vi "Create_Trajectory_Using_PathfinderSwerve_NAT.vi"() -> ()   [LabVIEW 2019]
uses:
  <vilib>/Rock Robotics/WPI/ThirdParty/JAS_Junk/JaciPathFinderLib/VIs/Waypoint.ctl
  <vilib>/Rock Robotics/WPI/ThirdParty/JAS_Junk/TrajLib/TRAJ_STATE.ctl
  <vilib>/Rock Robotics/WPI/ThirdParty/JAS_Junk/TrajLib/POSE2D.ctl
  <vilib>/Rock Robotics/WPI/ThirdParty/JAS_Junk/TrajLib/TRANSLATION2D.ctl
  <vilib>/Rock Robotics/WPI/ThirdParty/JAS_Junk/TrajLib/ROTATION2D.ctl
  <vilib>/Rock Robotics/WPI/ThirdParty/JAS_Junk/TrajLib/UTIL_PATHFINDER_CONFIG.ctl
  <vilib>/Rock Robotics/WPI/ThirdParty/JAS_Junk/TrajLib/DISPLAY_WAYPOINT.ctl
  <vilib>/Utility/inputDevices.llb/mouseAcquire.vi
  <vilib>/Rock Robotics/WPI/ThirdParty/JAS_Junk/JaciPathFinderLib/Pathfinder.lvlib
  <vilib>/Rock Robotics/WPI/ThirdParty/JAS_Junk/TrajLib/Trajectory_Library.lvlib
panel:
  out "Scrolling":i32
  out "Cursor Update Mode":i32=1
  out "Index":i32
  out "Angle":dbl
  out "CursIdx":i32
  in  "End Program":bool
  in  "Tab Control":T1(tab)
  in  "max_velocity":dbl=58.0
  in  "max_acceleration":dbl=65.0
  in  "max_jerk":dbl=70.0
  in  "wheelbase_width":dbl=20.866
  in  "Real max\n speed":dbl=65.0
  in  "wheelbase_depth":dbl=28.0
  in  "mode":u32(ring) items=["SWERVE_DEFAULT"]
  out "Position":cluster{dbl[], dbl[]}[](graph)
  in  "Remove Cursor":bool
  in  "Add Cursor":bool
  in  "Waypoints":T2[](array[typedef])=[{"x"=15.0, "y"=105.0, "angle"=-45.0}, {"x"=105.0, "y"=65.0, "angle"=0.0}, {"x"=210.0, "y"=106.0, "angle"=45.0}]
  in  "Path Results\ndT":dbl=0.02 format="%7.3f"
  in  "sample_count":i32=100000
  out "Path calculation error":errorcluster
  in  "Calculate\nPath":bool
  out "Complete,\nReady to \nSave file":bool
  out "Path \nSpeed > \nMax":bool
  out "max speed":dbl
  out "Path Data":cluster{dbl[], dbl[]}[](graph)
  out "Traj States\nSize":i32
  out "Trajectory States":T3[](array[typedef]) {"POSE"."ROTATION"."SIN" format="%13.4f"; "POSE"."ROTATION"."COS" format="%13.4f"; "POSE"."ROTATION"."VALUE" format="%13.4f"; "POSE"."TRANSLATION"."Y" format="%14.3f"; "POSE"."TRANSLATION"."X" format="%14.3f"}
  out "File Saved\nWithout\nError":bool
  in  "Trajectory Type":enum32{"Radio Selection 1", "Radio Selection 2"}(radio)
  out "File Creation\nError":errorcluster
  in  "Trajectory File Comment":string
  in  "Trajectory File Name":path
  in  "CreateCmdList":bool
  # "Create trajectory using \"Jaci's Pathfinder\"  (Display for swerve drive robot)"
  # "Instructions:\n----------------  \nThis utility will create a trajectory,, show the data on the various tabs, and optionally write a \"robot relative\" trajectory to a \nfile. To use this utility:\n\n1) Read all of these instructions!\n2) Define the Robot Data. on the \"Robot Data\" tab.\n3) Define the \"Path Definition\" on the \"Define / Create Trajectory\" tab.  These are the beginning and ending positions/headings, and \n     internal positions/headings.\n4) Define the time increment.  0.020 is chosen since that matches the normal robot loop time.\n5) Define \"sample count\".  This is an internal PathFinder variable.  Leaving the value as default should work correctly.  Making \n    the value a little smaller will speed the program up a little.\n6) Press the \"Calculate Path\".  If a good path was calculated it will be displayed on the \"Field Position tab, and the \"Complete, \n    Ready to Save\" indicator will light.  The path can be recalculated many times before performing any other action.\n\nAfter a Path has been calculated, the \"trajectory can be written to a file.  The absolute path is converted to a robot relative \ntrajectory.  To do this:\n1) Enter a comment to be included in the file.  Anything can be entered.\n2) Select the file name.\n3) Select the type of trajectory to save, absolute or relative.\n4) Press \"Create Trajectory File\"  If an error occurs it will be displayed in the File Creation Error indicator.\n\nNotes:\n---------\n- All the robot parameters, path, and field dimensions are in INCHES, and DEGREES.  The resulting trajectory is converted to \n   METERS, and RADIANS to match the rest of this library!\n- The pathfinder path generation logic doesn't account distribution of speed to the left and right wheels.  As a result the \n   maximum speed can be exceeded.If this happens, but Path Speed > Max light will light and Ready to Execute will not \n   light.  Lower the maximum speed in the Robot Data tab and recalulate the path.  (CURRENTLY THIS LOGIC IS NOT COMPLETE.)\n- 2019 playing field size - width: 26 ft 11.25 In = 323.25 in , length: 52 ft 5.25 in = 629.25 in  (I didn't verify this for the 2020 version.)"
  # "ROBOT DATA"
  # "INCHES/SEC"
  # "INCHES/SEC"
  # "INCHES/SEC^2"
  # "INCHES/SEC^3"
  # "Simulated robot wheelbase is: 20.866"
  # "INCHES"
  # "Simulated robot max speed is: 68.266"
  # "INCHES"
  # "SEC"
  # "PATH DEFINITION"
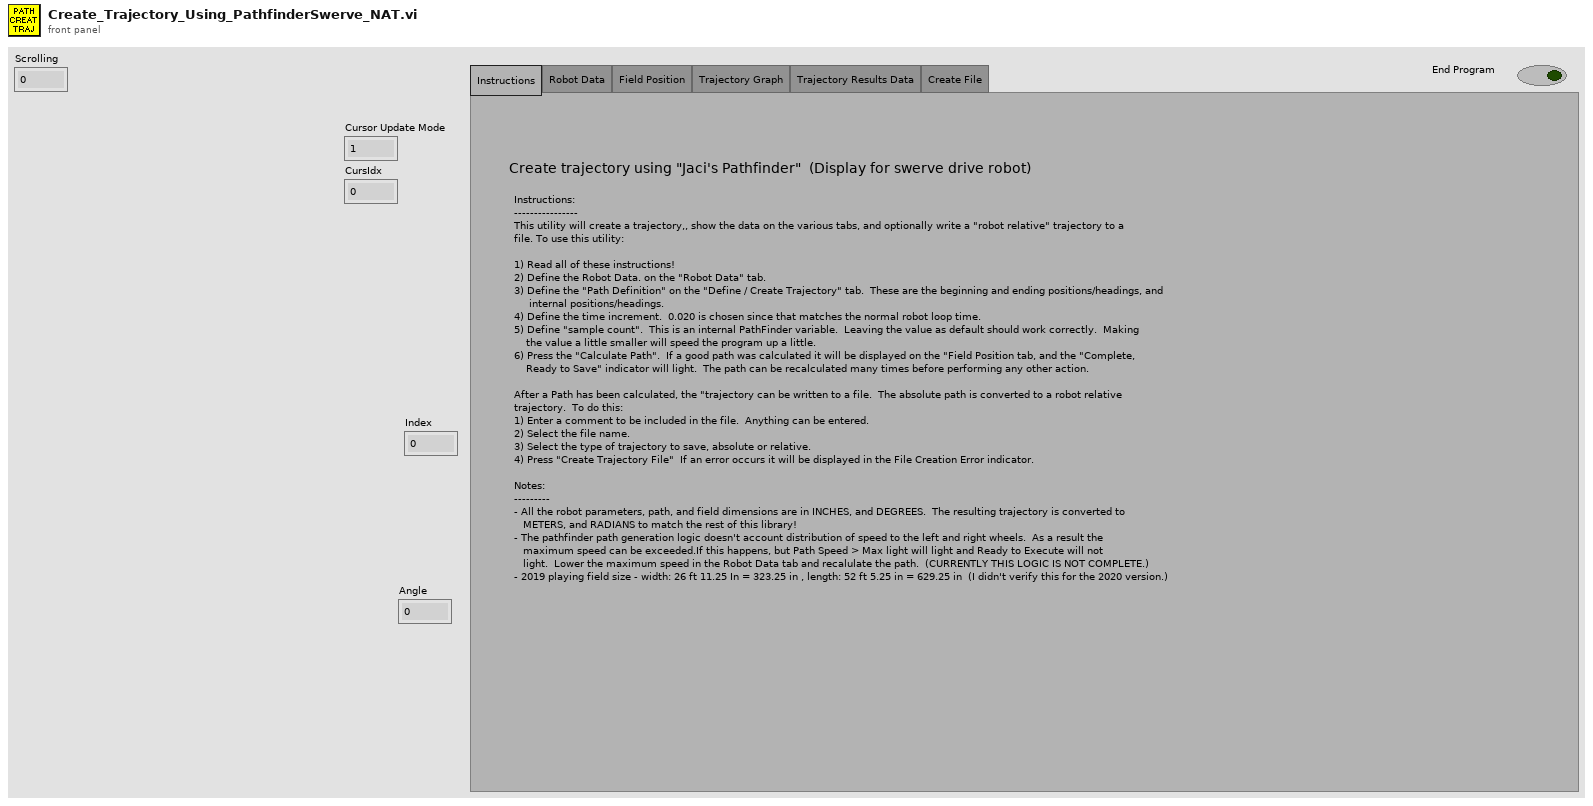
[diagram p1: front panel]
types:
  T1 = enum32{"Instructions", "Robot Data", "Field Position", "Trajectory Graph", "Trajectory Results Data", "Create File"}
  T2 = typedef "Pathfinder.lvlib/Waypoint.ctl" = cluster{"x":dbl, "y":dbl, "angle":dbl}
  T3 = typedef "Trajectory_Library.lvlib/TRAJ_STATE.ctl" = cluster{"TimeSeconds":dbl, "Velocity":dbl, "Acceleration":dbl, "POSE":T4, "Curvature":dbl}
  T4 = typedef "Trajectory_Library.lvlib/POSE2D.ctl" = cluster{"TRANSLATION":T5, "ROTATION":T6}
  T5 = typedef "Trajectory_Library.lvlib/TRANSLATION2D.ctl" = cluster{"X":dbl, "Y":dbl}
  T6 = typedef "Trajectory_Library.lvlib/ROTATION2D.ctl" = cluster{"VALUE":dbl, "COS":dbl, "SIN":dbl}
  T7 = cluster{"Name":string, "Color":u32, "Style":u8, "Point Style":u8, "Name Visible":bool, "Allow Drag":bool, "Cursor Mode":u32, "Plot":i32, "Index":i32, "Position":cluster{"X":dbl, "Y":dbl}, "X Scale":u32, "Y Scale":u32, "Watch Plots":i32[], "Watch All Plots":bool, "Plot Area":i32, "Label Offset":cluster{"X":dbl, "Y":dbl}}
  T8 = typedef "Trajectory_Library.lvlib/DISPLAY_WAYPOINT.ctl" = cluster{"X":dbl, "Y":dbl, "ANGLE":dbl}
  T9 = typedef "Trajectory_Library.lvlib/UTIL_PATHFINDER_CONFIG.ctl" = cluster{"PathfinderType - 0 tank 1 serve":i32, "PathMaxVelocity - inches per sec":dbl, "MaxAcceleration - inches per sec2":dbl, "MaxJerk--Inches per sec2":dbl, "TimeDelta-Seconds":dbl, "SampleCount":i32, "WheelbaseWidth-inches":dbl, "WheelbaseDepth-inches":dbl, "SwerveType":i32, "ActualMaxVelocity-inches per sec":dbl}
  T10 = typedef "LVCursorListTypeDef.ctl" = cluster{"Name":string, "Color":u32, "Style":u8, "Point Style":u8, "Name Visible":bool, "Allow Drag":bool, "Cursor Mode":u32, "Plot":i32, "Index":i32, "Position":cluster{"X":dbl, "Y":dbl}, "X Scale":u32, "Y Scale":u32, "Watch Plots":i32[], "Watch All Plots":bool, "Plot Area":i32, "Label Offset":cluster{"X":dbl, "Y":dbl}}[]
  T11 = cluster{"Horizontal":i32, "Vertical":i32, "Scrolling":i32}
  T12 = typedef "Trajectory_Library.lvlib/TRAJECTORY.ctl" = cluster{"TotalTImeSecs":dbl, "States":T3[]}
  T13 = typedef "Pathfinder.lvlib/Segment.ctl" = cluster{"dt":dbl, "x":dbl, "y":dbl, "position":dbl, "velocity":dbl, "acceleration":dbl, "jerk":dbl, "heading":dbl}
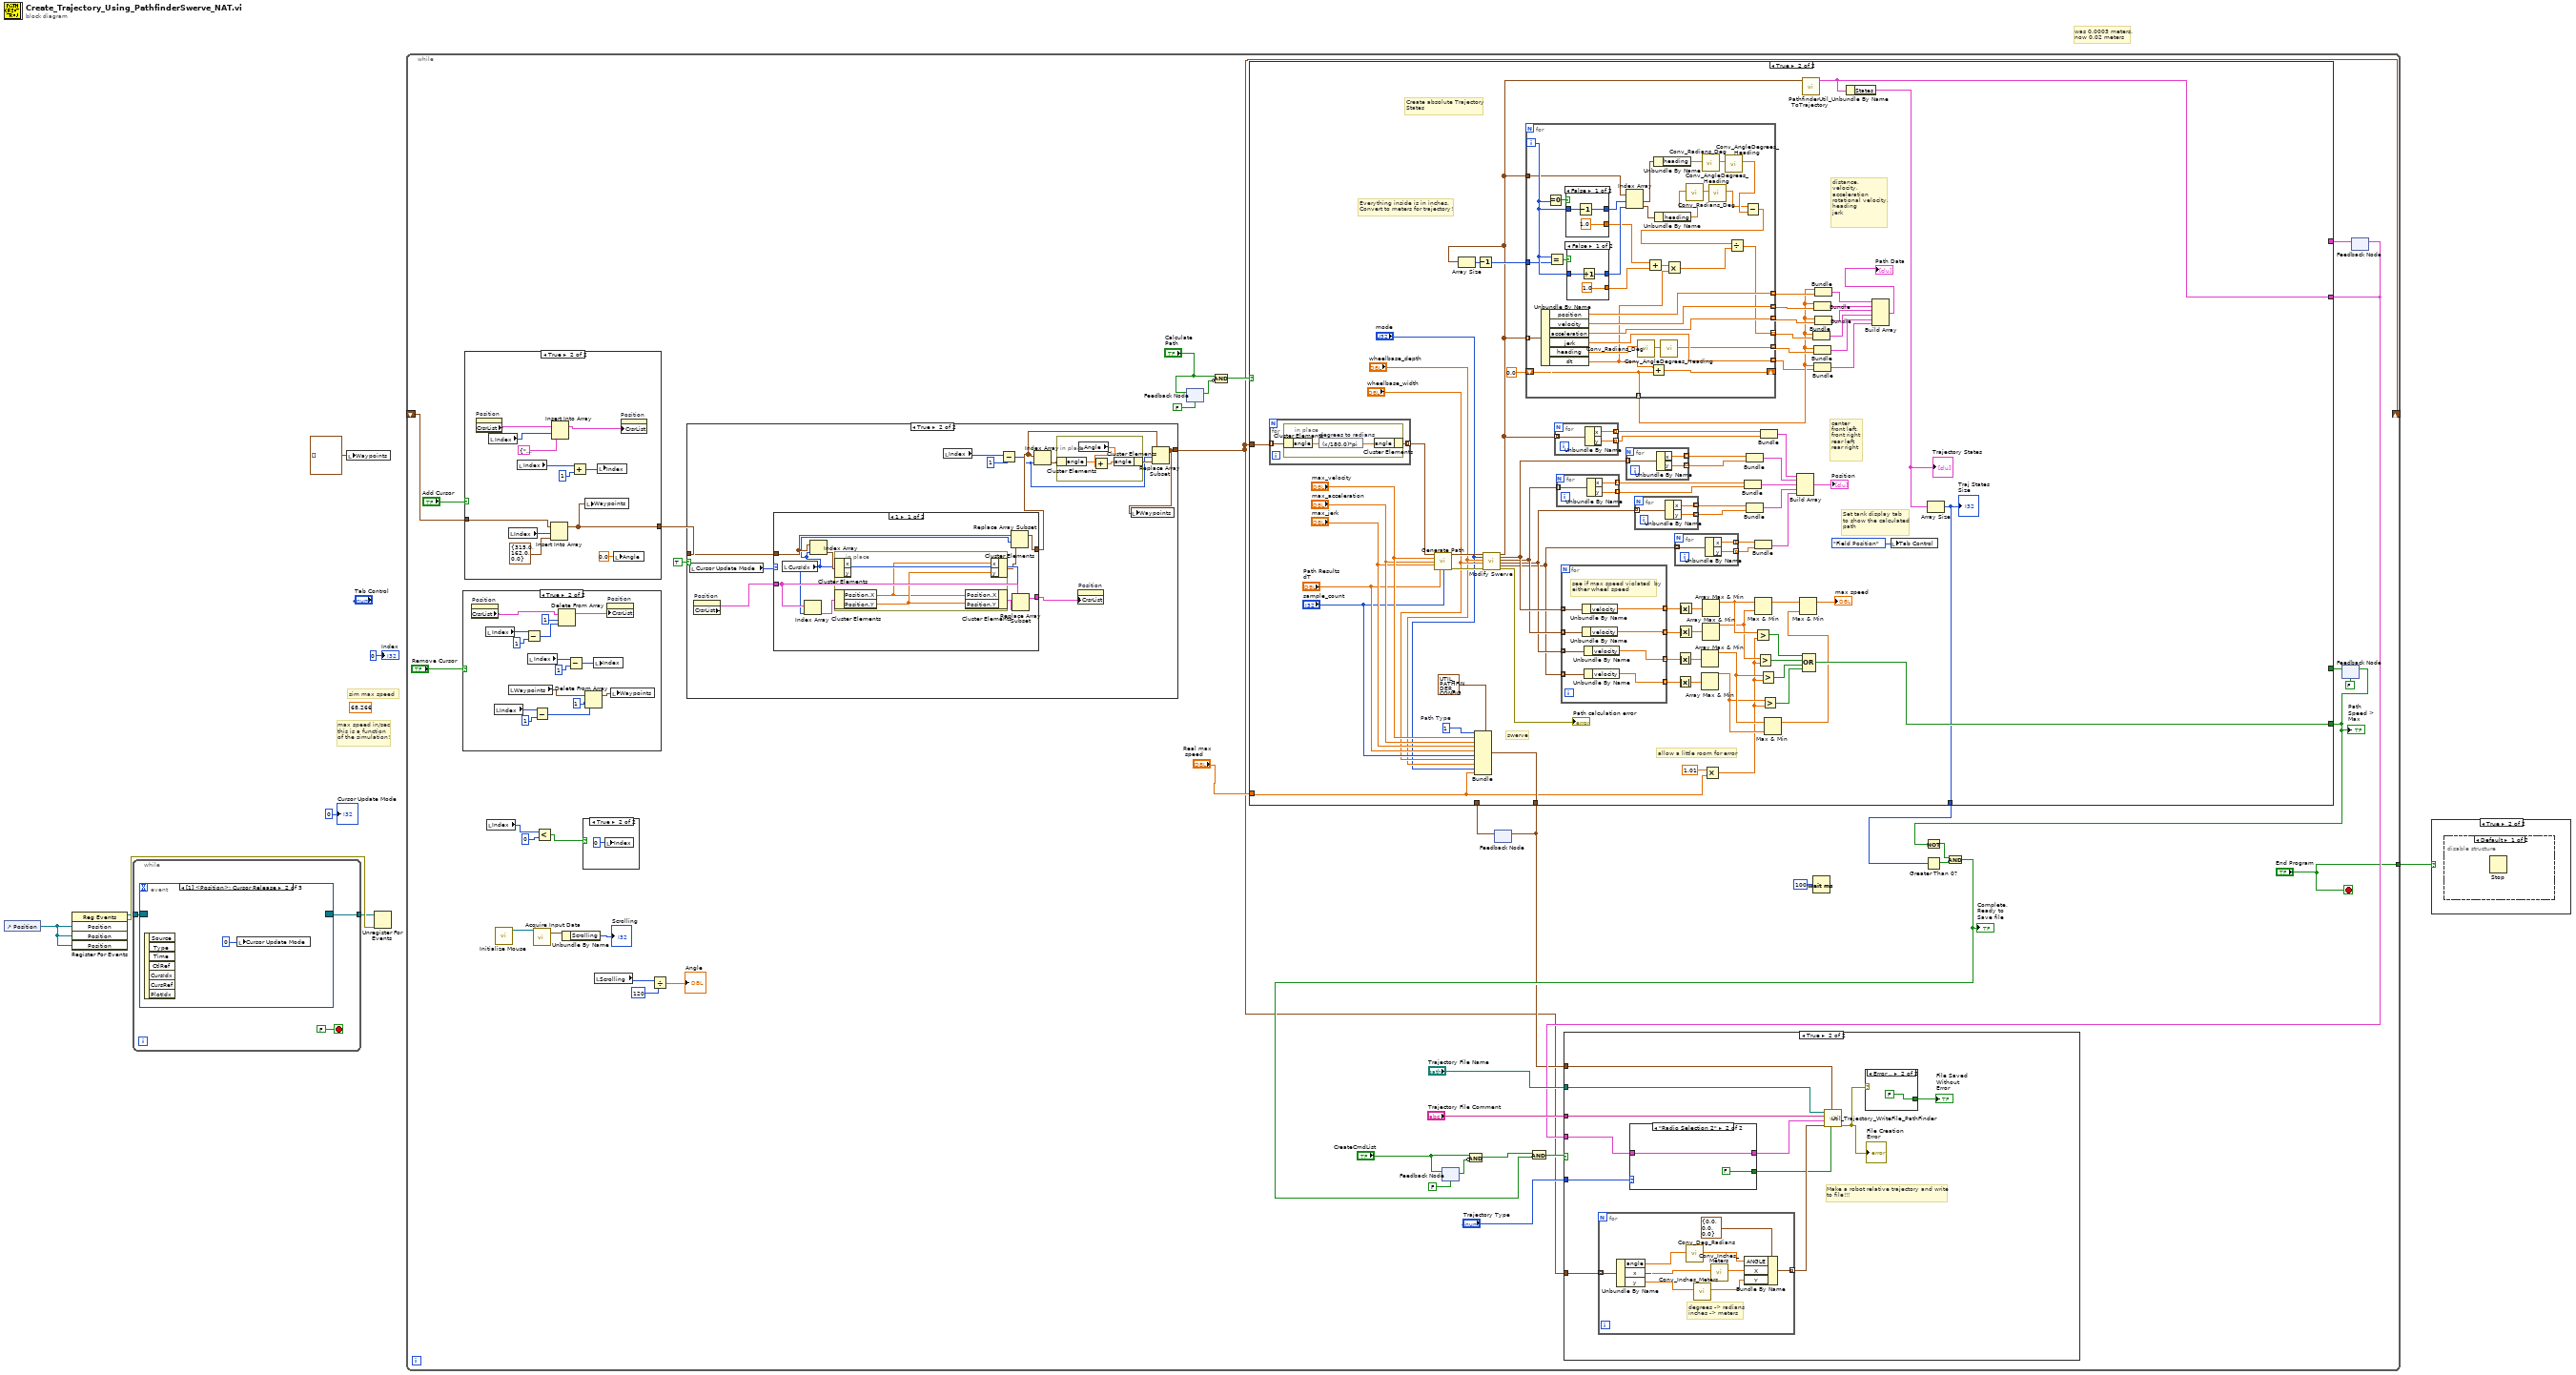
[diagram p0: block diagram]
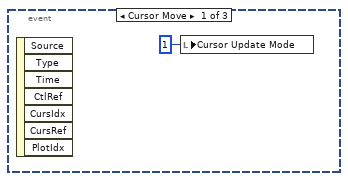
[diagram p2: hidden frame]
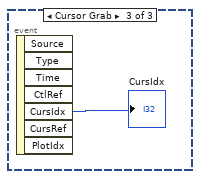
[diagram p3: hidden frame]
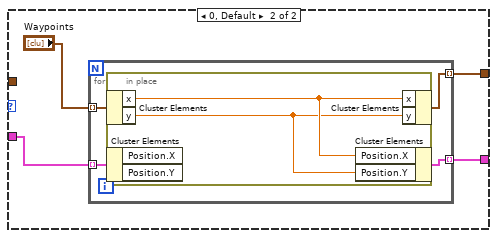
[diagram p6: hidden frame]
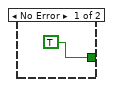
[diagram p10: hidden frame]
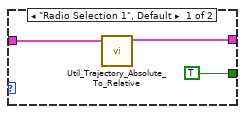
[diagram p11: hidden frame]
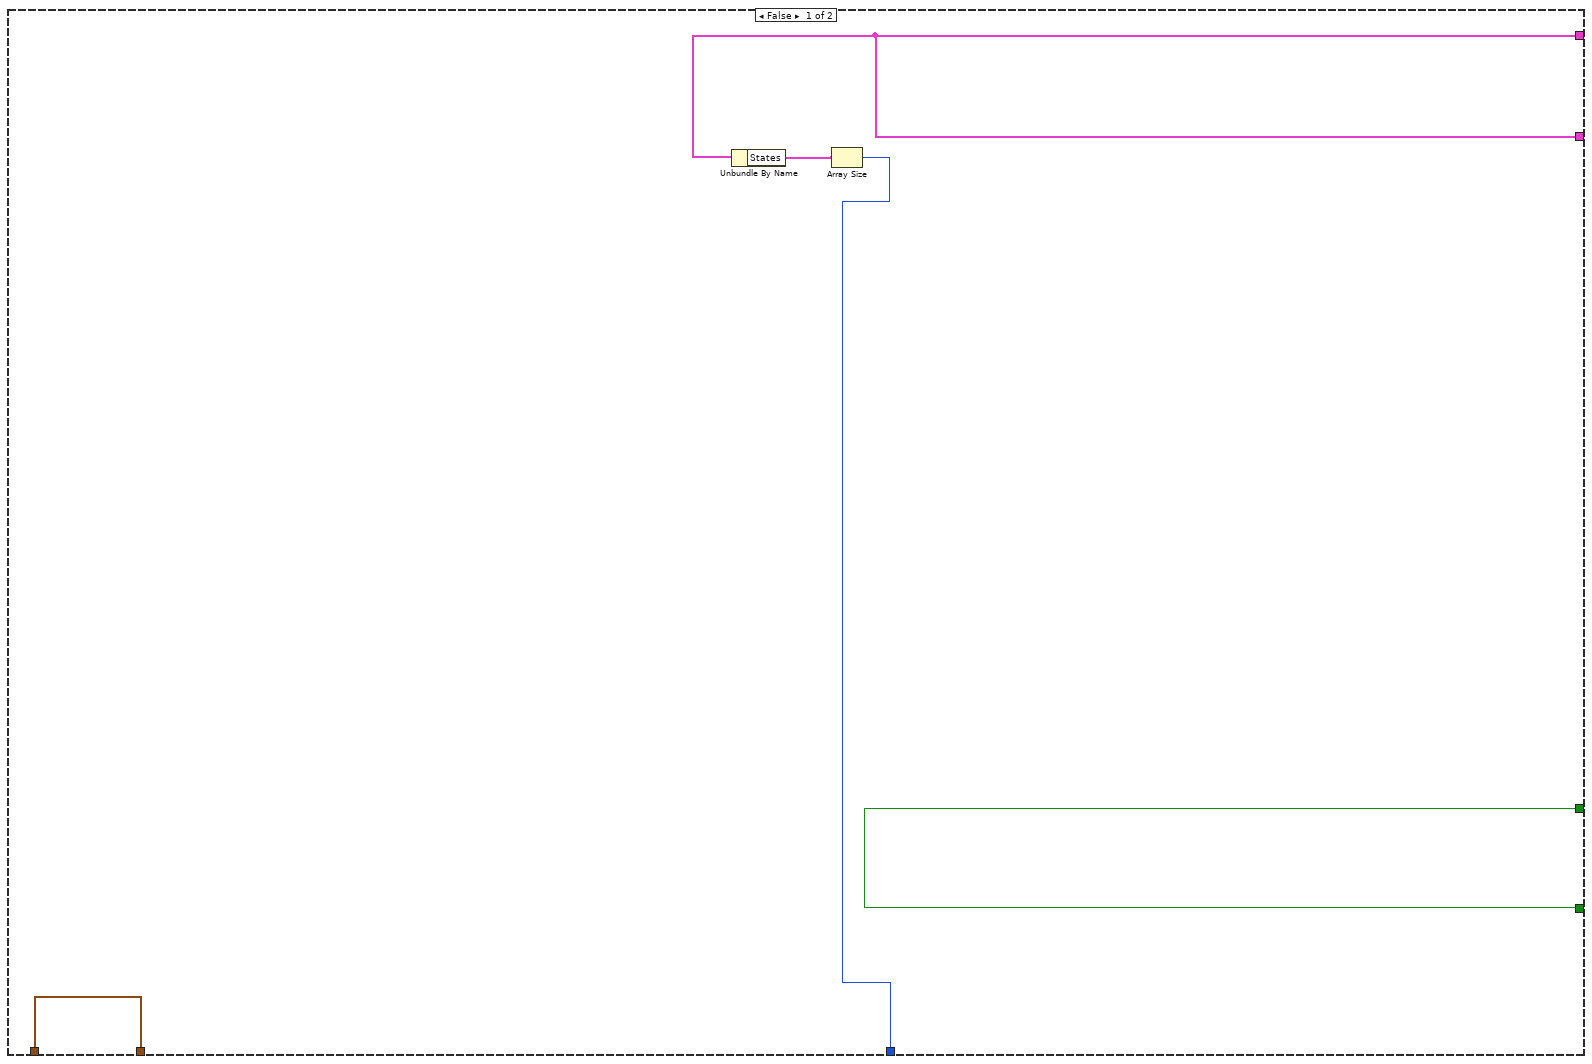
[diagram p12: hidden frame]
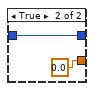
[diagram p13: hidden frame]
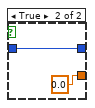
[diagram p14: hidden frame]
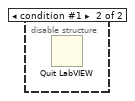
[diagram p16: hidden frame]
diagram:
  (unwired) 68.266 ("x")
  # "was 0.0003 meters.\nnow 0.02 meters"
  # "sim max speed"
  # "max speed in/sec\nthis is a function\nof the simulation!"
  n1 = control-ref of="Position"() -> (w2:refnum<vi>)
  n2 = register-events(w2, w2, w2) -> (reference out=w3:refnum<event-registration>, error out=w5:errorcluster)  [unwired: 2 in]
  n3 = while {
    tunnel: w3 -> [w11]
    tunnel: [w10] -> w4
    stop <- FALSE stop-if-true
    n4 = event shown="[1] <Position>: Cursor Release" {
      selector: w11 -> [_ _ _]
      dyn-events: [_ _ _] -> w10
      timeout: _ -> [_ _ _]
      event Cursor Move {
        n5 = event-data() -> ()  [unwired: 1 in, 7 out]
        n6 = local write "Cursor Update Mode"(1 ("Cursor Update Mode")) -> ()
      }
      event Cursor Release {
        n7 = event-data() -> ()  [unwired: 1 in, 7 out]
        n8 = local write "Cursor Update Mode"(0 ("Wapoint Update Mode")) -> ()
      }
      event Cursor Grab {
        n9 = event-data() -> ("CursIdx"=→"CursIdx":i32)  [unwired: 1 in, 6 out]
      }
    }
  }
  n10 = local write "Waypoints"(T2[] [] ("Waypoints")) -> ()
  n11 = Unregister For Events(event registration refnum=w4, error in=w5) -> ()  [unwired: 1 out]
  n12 = while {
    tunnel: ["End Program"] -> w8
    shift-right: [w25] -> _
    shift-left: _ -> [w24]
    stop <- "End Program" stop-if-true
    n13 = case shown="True" "Remove Cursor" {
      frame False {
      }
      frame True {
        n14 = property on="Position" class="XYGraph (strict)"() -> ("CrsrList"=w93:T10)  [unwired: 2 in, 2 out]
        n15 = local read "Index"() -> (w103:i32)
        n16 = local read "Index"() -> (w102:i32)
        n17 = local read "Waypoints"() -> (w96:T2[])
        n18 = Subtract(x=w103, y=1) -> (x-y=w100:i32)
        n19 = local read "Index"() -> (w106:i32)
        n20 = Subtract(x=w102, y=1) -> (x-y=w98:i32)
        n21 = Delete From Array(array=w93, length=1, index=w100) -> (array with subset deleted=w94:T10)  [unwired: 1 out]
        n22 = Subtract(x=w106, y=1) -> (x-y=w107:i32)
        n23 = Delete From Array(array=w96, length=1, index=w98) -> (array with subset deleted=w95:T2[])  [unwired: 1 out]
        n24 = local write "Index"(w107) -> ()
        n25 = property on="Position" class="XYGraph (strict)"("CrsrList"=w94) -> ()  [unwired: 2 in, 2 out]
        n26 = local write "Waypoints"(w95) -> ()
      }
    }
    n27 = case shown="True" "Add Cursor" {
      tunnel: w24 -> [w108 w114]
      tunnel: [w108 w112] -> w27
      frame False {
      }
      frame True {
        n28 = property on="Position" class="XYGraph (strict)"() -> ("CrsrList"=w109:T10)  [unwired: 2 in, 2 out]
        n29 = local read "Index"() -> (w120:i32)
        n30 = local read "Index"() -> (w116:i32)
        n31 = local read "Index"() -> (w118:i32)
        n32 = Insert Into Array(array=w114, index=w116, new element=T2 {"x"=315.0, "y"=162.0, "angle"=0.0} ("new element/subarray")) -> (w112:T2[])
        n33 = Insert Into Array(array=w109, index=w120, new element=T7 {"Name"="Cursor", "Color"=5635906, "Style"=4, "Point Style"=2, "Name Visible"=FALSE, "Allow Drag"=TRUE, "Cursor Mode"=0, "Plot"=0, "Index"=0, "Position"={"X"=315.0, "Y"=162.0}, "X Scale"=0, "Y Scale"=0, "Watch Plots"=[], "Watch All Plots"=FALSE, "Plot Area"=0, "Label Offset"={"X"=0.0, "Y"=0.0}} ("new element/subarray")) -> (w110:T10)
        n34 = Add(x=w118, y=1) -> (x+y=w117:i32)
        n35 = local write "Waypoints"(w112) -> ()
        n36 = local write "Index"(w117) -> ()
        n37 = local write "Angle"(0.0 ("Angle")) -> ()
        n38 = property on="Position" class="XYGraph (strict)"("CrsrList"=w110) -> ()  [unwired: 2 in, 2 out]
      }
    }
    n39 = local read "Index"() -> (w15:i32)
    n40 = call <vilib>:"Initialize Mouse.vi"() -> ("device ID"=w19:refnum<k1>)  [unwired: 10 in, 1 out]
    n41 = call-poly <vilib>:"Acquire Input Data.vi"("device ID"=w19) -> ("axis info"=w20:T11)  [unwired: 15 in, 3 out]
    n42 = Less?(x=w15, y=0) -> (x < y?=w17:bool)
    n43 = Unbundle By Name(w20) -> ("Scrolling"=→"Scrolling":i32)
    n44 = case shown="True" w17 {
      frame False {
      }
      frame True {
        n45 = local write "Index"(0 ("Index")) -> ()
      }
    }
    n46 = local read "Scrolling"() -> (w23:i32)
    n47 = Divide(x=w23, y=120) -> (x/y=→"Angle":dbl)
    n48 = case shown="True" TRUE {
      tunnel: w27 -> [w57 w67]
      tunnel: [w57 w60] -> w25
      frame False {
      }
      frame True {
        n49 = local read "Cursor Update Mode"() -> (w68:i32)
        n50 = property on="Position" class="XYGraph (strict)"() -> ("CrsrList"=w58:T10)  [unwired: 2 in, 2 out]
        n51 = case shown="1" w68 {
          tunnel: w58 -> [w75 w86]
          tunnel: w67 -> [w78 _]
          tunnel: [w77 w85] -> w63
          tunnel: [w73 w84] -> w59
          frame 1 {
            n52 = local read "CursIdx"() -> (w74:i32)
            n53 = Index Array(array=w75, index=w74) -> (element=w80:T7)
            n54 = Index Array(array=w78, index=w74) -> (element=w79:T2)
            n55 = in-place {
              n56 = in-place-cluster #1(w79) -> ()  [unwired: 2 out]
              n57 = in-place-cluster #2(w80) -> ("Position.X"=w81:dbl, "Position.Y"=w82:dbl)
              n58 = in-place-cluster #2("Position.X"=w81, "Position.Y"=w82) -> (w76:T7)
              n59 = in-place-cluster #1("x"=w81, "y"=w82) -> (w72:T2)
            }
            n60 = Replace Array Subset(array=w78, new element=w72, index=w74) -> (w77:T2[])
            n61 = Replace Array Subset(array=w75, new element=w76, index=w74) -> (w73:T10)
          }
          frame 0, Default {
            n62 = for {
              tunnel: w86 -> [w90] mode=indexing
              tunnel: "Waypoints" -> [w89] mode=indexing
              tunnel: [w88] -> w85 mode=indexing
              tunnel: [w87] -> w84 mode=indexing
              n63 = in-place {
                n64 = in-place-cluster #3(w89) -> ("x"=w92:dbl, "y"=w91:dbl)
                n65 = in-place-cluster #4(w90) -> ()  [unwired: 2 out]
                n66 = in-place-cluster #4("Position.X"=w92, "Position.Y"=w91) -> (w87:T7)
                n67 = in-place-cluster #3("x"=w92, "y"=w91) -> (w88:T2)
              }
            }
          }
        }
        n68 = local read "Index"() -> (w62:i32)
        n69 = Subtract(x=w62, y=1) -> (x-y=w61:i32)
        n70 = Index Array(array=w63, index=w61) -> (element=w64:T2)
        n71 = in-place {
          n72 = in-place-cluster #5(w64) -> ("angle"=w71:dbl)
          n73 = local read "Angle"() -> (w70:dbl)
          n74 = Add(x=w70, y=w71) -> (x+y=w69:dbl)
          n75 = in-place-cluster #5("angle"=w69) -> (w66:T2)
        }
        n76 = property on="Position" class="XYGraph (strict)"("CrsrList"=w59) -> ()  [unwired: 2 in, 2 out]
        n77 = Replace Array Subset(array=w63, new element=w66, index=w61) -> (w60:T2[])
        n78 = local write "Waypoints"(w60) -> ()
      }
    }
    n79 = feedback #6(FALSE ("CreateCmdList")) -> (w38:bool)
    n80 = feedback-in #6("Calculate\nPath") -> ()
    n81 = Compound Arithmetic op=AND("Calculate\nPath", invert w38) -> (w35:bool)
    n82 = feedback #7(FALSE ("CreateCmdList")) -> (w41:bool)
    n83 = feedback-in #7("CreateCmdList") -> ()
    n84 = Compound Arithmetic op=AND("CreateCmdList", invert w41) -> (w40:bool)
    n85 = feedback #8() -> (w30:T9)  [unwired: 1 in]
    n86 = Wait (ms)(milliseconds to wait=u32 100) -> ()  [unwired: 1 out]
    n87 = feedback #9(FALSE) -> (w53:bool)
    n88 = feedback #10() -> (w49:T12)  [unwired: 1 in]
    n89 = case shown="True" w35 {
      tunnel: "Real max\n speed" -> [_ w154]
      tunnel: [w152 w219] -> w50
      tunnel: w53 -> [w152 _]
      tunnel: w25 -> [_ w218]
      tunnel: [w149 w198] -> w44
      tunnel: w49 -> [w149 _]
      tunnel: [w151 w212] -> w43
      tunnel: [w148 w157] -> w31
      tunnel: w30 -> [w148 _]
      frame False {
        n90 = Unbundle By Name(w149) -> ("States"=w150:T3[])
        n91 = Array Size(array=w150) -> (size(s)=w151:i32)
      }
      frame True {
        w166 = 1  # Path Type
        # "allow a little room for error"
        # "center\nfront left,\nfront right\nrear left\nrear right"
        # "distance,\nvelocity,\nacceleration\nrotational velocity,\nheading\njerk"
        # "swerve"
        # "Everything inside is in inches.\nConvert to meters for trajectory!"
        # "Create absolute Trajectory\nStates"
        # "Set tank display tab\nto show the calculated\npath"
        n92 = for {
          tunnel: w218 -> [w249] mode=indexing
          tunnel: [w248] -> w231 mode=indexing
          n93 = in-place {
            n94 = in-place-cluster #11(w249) -> ("angle"=w251:dbl)
            n95 = expression code="(x/180.0)*pi" "degrees to radians"(w251) -> (w250:dbl)
            n96 = in-place-cluster #11("angle"=w250) -> (w248:T2)
          }
        }
        n97 = call <vilib>:"Generate Path.vi"("path"=w231, "max_velocity"="max_velocity", "max_acceleration"="max_acceleration", "max_jerk"="max_jerk", "dt (.001)"="Path Results\ndT", "sample_count (100000)"="sample_count") -> ("Segments"=w232:T13[], "error out"=w188:errorcluster)  [unwired: 8 in]
        n98 = Bundle(cluster=T9 {"PathfinderType - 0 tank 1 serve"=0, "PathMaxVelocity - inches per sec"=0.0, "MaxAcceleration - inches per sec2"=0.0, "MaxJerk--Inches per sec2"=0.0, "TimeDelta-Seconds"=0.0, "SampleCount"=0, "WheelbaseWidth-inches"=0.0, "WheelbaseDepth-inches"=0.0, "SwerveType"=0, "ActualMaxVelocity-inches per sec"=0.0} ("UTIL_PATHFINDER_CONFIG"), "PathfinderType - 0 tank 1 serve"=w166, "PathMaxVelocity - inches per sec"="max_velocity", "MaxAcceleration - inches per sec2"="max_acceleration", "MaxJerk--Inches per sec2"="max_jerk", "TimeDelta-Seconds"="Path Results\ndT", "SampleCount"="sample_count", "WheelbaseWidth-inches"="wheelbase_width", "WheelbaseDepth-inches"="wheelbase_depth", "SwerveType"="mode", "ActualMaxVelocity-inches per sec"=w154) -> (w157:T9)
        n99 = call <vilib>:"Modify Swerve.vi"("Original"=w232, "mode"="mode", "wheelbase_depth"="wheelbase_depth", "wheelbase_width"="wheelbase_width", "error in"=w188) -> ("Original"=w189:T13[], "front_left out"=w172:T13[], "front_right out"=w171:T13[], "back_left out"=w170:T13[], "back_right out"=w169:T13[], "error out"=→"Path calculation error":errorcluster)  [unwired: 9 in]
        n100 = Array Size(array=w189) -> (size(s)=w191:i32)
        n101 = Decrement(x=w191) -> (x-1=w190:i32)
        n102 = for {
          tunnel: w189 -> [w292] mode=indexing
          shift-right: [w290] -> _
          shift-left: 0.0 -> [w291]
          tunnel: [w291] -> w194 mode=indexing
          tunnel: [w283] -> w195 mode=indexing
          tunnel: [w289] -> w193 mode=indexing
          tunnel: [w288] -> w203 mode=indexing
          tunnel: [w287] -> w202 mode=indexing
          tunnel: [w286] -> w197 mode=indexing
          tunnel: [w269] -> w196 mode=indexing
          tunnel: w189 -> [w275]
          tunnel: w190 -> [w268]
          i -> [w280]
          n103 = Unbundle By Name(w292) -> ("position"=w286:dbl, "velocity"=w287:dbl, "acceleration"=w288:dbl, "jerk"=w289:dbl, "heading"=w285:dbl, "dt"=w271:dbl)
          n104 = Equal To 0?(x=w280) -> (x = 0?=w282:bool)
          n105 = Equal?(x=w280, y=w268) -> (x = y?=w281:bool)
          n106 = case shown="False" w282 {
            tunnel: w280 -> [w300 w301]
            tunnel: [1.0 0.0] -> w272
            tunnel: [w298 w301] -> w277
            frame False {
              n107 = Decrement(x=w300) -> (x-1=w298:i32)
            }
            frame True {
            }
          }
          n108 = case shown="False" w281 {
            tunnel: [1.0 0.0] -> w273
            tunnel: w280 -> [w294 w296]
            tunnel: [w293 w296] -> w276
            frame False {
              n109 = Increment(x=w294) -> (x+1=w293:i32)
            }
            frame True {
            }
          }
          n110 = Index Array(array=w275, index #1=w277, index #2=w276) -> (element #1=w279:T13, element #2=w278:T13)
          n111 = call <vilib>:"Conv_Radians_Deg.vi"("Radians"=w285) -> ("Degrees"=w284:dbl)  [unwired: 10 in]
          n112 = Add(x=w272, y=w273) -> (x+y=w274:dbl)
          n113 = Add(x=w271, y=w291) -> (x+y=w290:dbl)
          n114 = Unbundle By Name(w279) -> ("heading"=w265:dbl)
          n115 = Unbundle By Name(w278) -> ("heading"=w263:dbl)
          n116 = call <vilib>:"Conv_AngleDegrees_Heading.vi"("Degrees"=w284) -> ("Heading Degrees"=w283:dbl)  [unwired: 10 in]
          n117 = Multiply(x=w274, y=w271) -> (x*y=w270:dbl)
          n118 = call <vilib>:"Conv_Radians_Deg.vi"("Radians"=w263) -> ("Degrees"=w262:dbl)  [unwired: 10 in]
          n119 = call <vilib>:"Conv_Radians_Deg.vi"("Radians"=w265) -> ("Degrees"=w266:dbl)  [unwired: 10 in]
          n120 = call <vilib>:"Conv_AngleDegrees_Heading.vi"("Degrees"=w262) -> ("Heading Degrees"=w261:dbl)  [unwired: 10 in]
          n121 = call <vilib>:"Conv_AngleDegrees_Heading.vi"("Degrees"=w266) -> ("Heading Degrees"=w264:dbl)  [unwired: 10 in]
          n122 = Subtract(x=w261, y=w264) -> (x-y=w267:dbl)
          n123 = Divide(x=w267, y=w270) -> (x/y=w269:dbl)
        }
        n124 = for {
          tunnel: w189 -> [w254] mode=indexing
          tunnel: [w253] -> w228 mode=indexing
          tunnel: [w252] -> w229 mode=indexing
          n125 = Unbundle By Name(w254) -> ("x"=w253:dbl, "y"=w252:dbl)
        }
        n126 = for {
          tunnel: w171 -> [w257] mode=indexing
          tunnel: [w256] -> w224 mode=indexing
          tunnel: [w255] -> w225 mode=indexing
          n127 = Unbundle By Name(w257) -> ("x"=w256:dbl, "y"=w255:dbl)
        }
        n128 = for {
          tunnel: w172 -> [w247] mode=indexing
          tunnel: w171 -> [w246] mode=indexing
          tunnel: [w245] -> w217 mode=indexing
          tunnel: [w244] -> w215 mode=indexing
          tunnel: w169 -> [w243] mode=indexing
          tunnel: w170 -> [w242] mode=indexing
          tunnel: [w241] -> w185 mode=indexing
          tunnel: [w240] -> w184 mode=indexing
          # "see if max speed violated  by\neither wheel speed"
          n129 = Unbundle By Name(w247) -> ("velocity"=w245:dbl)
          n130 = Unbundle By Name(w246) -> ("velocity"=w244:dbl)
          n131 = Unbundle By Name(w242) -> ("velocity"=w241:dbl)
          n132 = Unbundle By Name(w243) -> ("velocity"=w240:dbl)
        }
        n133 = for {
          tunnel: w172 -> [w260] mode=indexing
          tunnel: [w259] -> w222 mode=indexing
          tunnel: [w258] -> w223 mode=indexing
          n134 = Unbundle By Name(w260) -> ("x"=w259:dbl, "y"=w258:dbl)
        }
        n135 = for {
          tunnel: w170 -> [w239] mode=indexing
          tunnel: [w238] -> w176 mode=indexing
          tunnel: [w237] -> w175 mode=indexing
          n136 = Unbundle By Name(w239) -> ("x"=w238:dbl, "y"=w237:dbl)
        }
        n137 = for {
          tunnel: w169 -> [w236] mode=indexing
          tunnel: [w235] -> w174 mode=indexing
          tunnel: [w234] -> w173 mode=indexing
          n138 = Unbundle By Name(w236) -> ("x"=w235:dbl, "y"=w234:dbl)
        }
        n139 = Absolute Value(x=w185) -> (abs(x)=w187:dbl[])
        n140 = Absolute Value(x=w184) -> (abs(x)=w186:dbl[])
        n141 = Absolute Value(x=w217) -> (abs(x)=w216:dbl[])
        n142 = Absolute Value(x=w215) -> (abs(x)=w214:dbl[])
        n143 = Array Max & Min(array=w187) -> (max value=w181:dbl)  [unwired: 3 out]
        n144 = Array Max & Min(array=w186) -> (max value=w180:dbl)  [unwired: 3 out]
        n145 = Array Max & Min(array=w216) -> (max value=w211:dbl)  [unwired: 3 out]
        n146 = Array Max & Min(array=w214) -> (max value=w210:dbl)  [unwired: 3 out]
        n147 = Multiply(x=1.01, y=w154) -> (x*y=w155:dbl)
        n148 = Bundle(w224, w225) -> (w226:cluster{dbl[], dbl[]})  [unwired: 1 in]
        n149 = Bundle(w222, w223) -> (w227:cluster{dbl[], dbl[]})  [unwired: 1 in]
        n150 = Bundle(w176, w175) -> (w168:cluster{dbl[], dbl[]})  [unwired: 1 in]
        n151 = Bundle(w174, w173) -> (w167:cluster{dbl[], dbl[]})  [unwired: 1 in]
        n152 = Max & Min(x=w211, y=w210) -> (max(x,y)=w178:dbl)  [unwired: 1 out]
        n153 = Greater?(x=w211, y=w155) -> (0:w220:bool)
        n154 = Greater?(x=w210, y=w155) -> (0:w213:bool)
        n155 = Greater?(x=w181, y=w155) -> (0:w183:bool)
        n156 = Bundle(w228, w229) -> (w230:cluster{dbl[], dbl[]})  [unwired: 1 in]
        n157 = Greater?(x=w180, y=w155) -> (0:w182:bool)
        n158 = Max & Min(x=w181, y=w180) -> (max(x,y)=w179:dbl)  [unwired: 1 out]
        n159 = Build Array(w230, w227, w226, w168, w167) -> (→"Position":cluster{dbl[], dbl[]}[])
        n160 = Max & Min(x=w178, y=w179) -> (max(x,y)=→"max speed":dbl)  [unwired: 1 out]
        n161 = call <vilib>:"PathfinderUtil_ToTrajectory.vi"("Pathfinder Path"=w189) -> ("TRAJECTORY"=w198:T12)  [unwired: 10 in]
        n162 = Compound Arithmetic op=OR(w220, w213, w183, w182) -> (w219:bool)
        n163 = Bundle(w194, w196) -> (w206:cluster{dbl[], dbl[]})  [unwired: 1 in]
        n164 = Bundle(w194, w195) -> (w205:cluster{dbl[], dbl[]})  [unwired: 1 in]
        n165 = Bundle(w194, w202) -> (w208:cluster{dbl[], dbl[]})  [unwired: 1 in]
        n166 = Bundle(w194, w193) -> (w192:cluster{dbl[], dbl[]})  [unwired: 1 in]
        n167 = Bundle(w194, w197) -> (w209:cluster{dbl[], dbl[]})  [unwired: 1 in]
        n168 = Bundle(w194, w203) -> (w207:cluster{dbl[], dbl[]})  [unwired: 1 in]
        n169 = Unbundle By Name(w198) -> ("States"=w200:T3[])
        "Trajectory States" <- w200
        n170 = Build Array(w209, w208, w207, w206, w205, w192) -> (→"Path Data":cluster{dbl[], dbl[]}[])
        n171 = local write "Tab Control"(T1."Field Position" ("Tab Control")) -> ()
        n172 = Array Size(array=w200) -> (size(s)=w212:i32)
        "Traj States\nSize" <- w212
      }
    }
    "Path \nSpeed > \nMax" <- w50
    n173 = feedback-in #8(w31) -> ()
    n174 = Not(x=w50) -> (.not. x?=w51:bool)
    n175 = Greater Than 0?(x=w43) -> (x > 0?=w52:bool)
    n176 = And(x=w51, y=w52) -> (x .and. y?=w45:bool)
    "Complete,\nReady to \nSave file" <- w45
    n177 = And(x=w40, y=w45) -> (x .and. y?=w46:bool)
    n178 = case shown="True" w46 {
      tunnel: "Trajectory File Name" -> [_ w131]
      tunnel: "Trajectory File Comment" -> [_ w130]
      tunnel: w44 -> [_ w126]
      tunnel: w25 -> [_ w129]
      tunnel: "Trajectory Type" -> [_ w125]
      tunnel: w31 -> [_ w121]
      frame False {
      }
      frame True {
        # "Make a robot relative trajectory and write\nto file!!!"
        n179 = for {
          tunnel: w129 -> [w147] mode=indexing
          tunnel: [w146] -> w128 mode=indexing
          # "degrees -> radians\ninches -> meters"
          n180 = Unbundle By Name(w147) -> ("angle"=w140:dbl, "x"=w145:dbl, "y"=w143:dbl)
          n181 = call <vilib>:"Conv_Deg_Radians.vi"("Degress"=w140) -> ("Radians"=w141:dbl)  [unwired: 10 in]
          n182 = call <vilib>:"Conv_Inches_Meters.vi"("INCH"=w143) -> ("Meters"=w142:dbl)  [unwired: 10 in]
          n183 = call <vilib>:"Conv_Inches_Meters.vi"("INCH"=w145) -> ("Meters"=w144:dbl)  [unwired: 10 in]
          n184 = Bundle By Name(cluster=T8 {"X"=0.0, "Y"=0.0, "ANGLE"=0.0} ("UTIL_WAYPOINT"), "ANGLE"=w141, "X"=w144, "Y"=w142) -> (w146:T8)
        }
        n185 = case shown="\"Radio Selection 2\"" w125 {
          tunnel: w126 -> [w136 w138]
          tunnel: [w135 w138] -> w127
          tunnel: [TRUE FALSE] -> w122
          frame "Radio Selection 1", Default {
            n186 = call <vilib>:"Util_Trajectory_Absolute_To_Relative.vi"("absTRAJECTORY"=w136) -> ("outputRelativeTRAJECTORY"=w135:T12)  [unwired: 10 in]
          }
          frame "Radio Selection 2" {
          }
        }
        n187 = call <vilib>:"Util_Trajectory_WriteFile_PathFinder.vi"("Trajectory Is Relative"=w122, "UTIL_PATHFINDER_CONFIG"=w121, "UtilityWayPoints"=w128, "TRAJECTORY"=w127, "Comment"=w130, "Trajectory File Name"=w131) -> ("error out"=w124:errorcluster)  [unwired: 5 in]
        "File Creation\nError" <- w124
        n188 = case shown="Error .." w124 {
          tunnel: [TRUE ("File Saved\nWithout\nError") FALSE ("File Saved\nWithout\nError")] -> w123
          frame No Error {
          }
          frame Error {
          }
        }
        "File Saved\nWithout\nError" <- w123
      }
    }
    n189 = feedback-in #9(w50) -> ()
    n190 = feedback-in #10(w44) -> ()
  }
  n191 = case shown="True" w8 {
    frame False {
    }
    frame True {
      n192 = disable-structure shown="Default" {
        frame condition #0 (active) {
          n193 = Stop() -> ()  [unwired: 1 in]
        }
        frame condition #1 {
          n194 = Quit LabVIEW() -> ()  [unwired: 1 in]
        }
      }
    }
  }
  "Index" <- 0 ("Index")
  "Cursor Update Mode" <- 0 ("Cursor Update Mode")
